vi "Build Messgenger.vi"(7 "Messenger Factory in":refnum<class "Messenger Factory.lvclass">, 8 "error in (no error)":errorcluster, 10 "System Modules Factory In":refnum<class "System Modules Factory.lvclass">, 11 "Root Actor In":refnum<class "Root Actor.lvclass">) -> (0 "error out":errorcluster, 3 "Root Actor Out":refnum<class "Root Actor.lvclass">, 5 "Messenger Factory out":refnum<class "Messenger Factory.lvclass">)   [LabVIEW 2024, in "Messenger Factory.lvclass"]
uses:
  Messenger Factory.lvclass
  Actor/Root Actor/Root Actor.lvclass
  System Modules Factory/System Modules Factory.lvclass
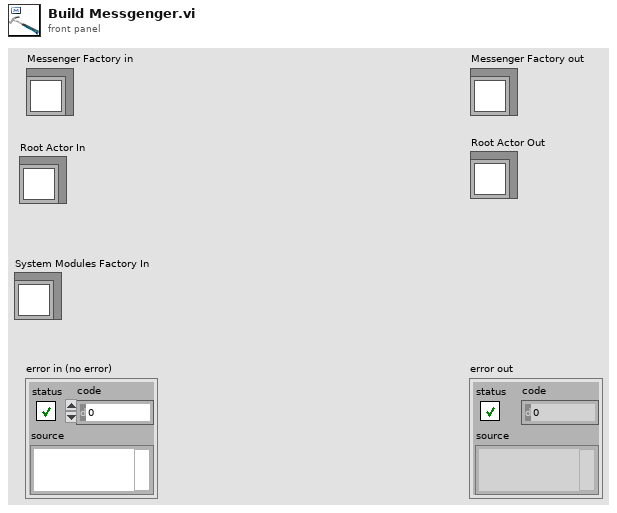
[diagram p1: front panel]
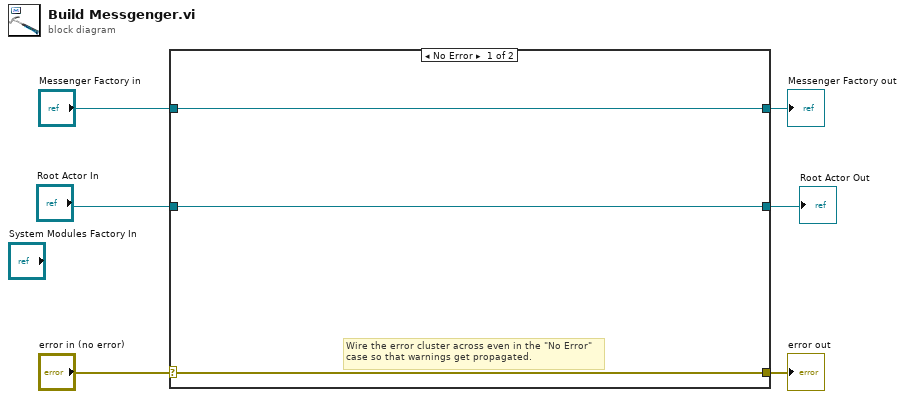
[diagram p0: block diagram]
diagram:
  n1 = case shown="No Error" "error in (no error)" {
    selector: "error in (no error)" -> [w8 w12]
    tunnel: [w8 w12] -> w5
    tunnel: [w9 w11] -> w3
    tunnel: "Messenger Factory in" -> [w9 w11]
    tunnel: [w7 w10] -> w1
    tunnel: "Root Actor In" -> [w7 w10]
    frame No Error {
      # "Wire the error cluster across even in the \"No Error\"\ncase so that warnings get propagated."
    }
    frame Error {
    }
  }
  "error out" <- w5
  "Messenger Factory out" <- w3
  "Root Actor Out" <- w1
